vi "position_initialize.vi"(6 "Axis in":i32, 7 "New target position (units)":dbl, 9 "Velocity value (units/s)":dbl, 10 "Timeout (ms)":u32, 11 "SerialPort":u8) -> (3 "VISA Refnum out":refnum<visa-resource-name>)   [LabVIEW 2021]
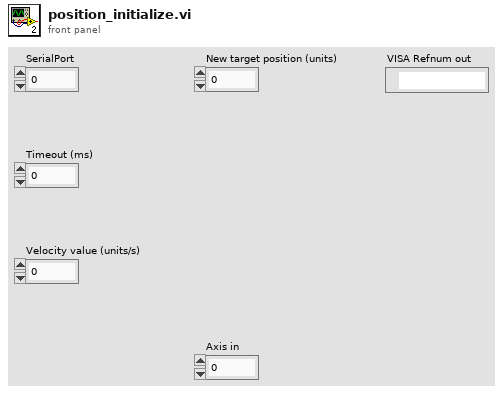
[diagram p1: front panel]
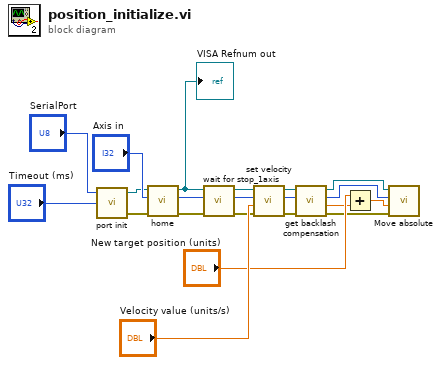
[diagram p0: block diagram]
diagram:
  n1 = call <userlib>:"port init.vi"("Timeout (ms)"="Timeout (ms)", "SerialPort"="SerialPort") -> ("error out"=w16:errorcluster, "Visa Handle"=w17:refnum<visa-resource-name>)  [unwired: 2 in]
  n2 = call <userlib>:"home.vi"("error in"=w16, "Axis in"="Axis in", "VISA Handle in"=w17) -> ("error out"=w13:errorcluster, "Axis out"=w14:i32, "VISA Handle out"=w15:refnum<visa-resource-name>)  [unwired: 3 in, 1 out]
  "VISA Refnum out" <- w15
  n3 = call <userlib>:"wait for stop_1axis.vi"("error in"=w13, "Axis in"=w14, "VISA Handle in"=w15) -> ("error out"=w10:errorcluster, "Axis out"=w11:i32, "VISA Handle out"=w12:refnum<visa-resource-name>)  [unwired: 3 in, 1 out]
  n4 = call <userlib>:"set velocity.vi"("error in"=w10, "Velocity value (units/s)"="Velocity value (units/s)", "Axis in"=w11, "VISA Handle in"=w12) -> ("error out"=w5:errorcluster, "Axis out"=w6:i32, "VISA Handle out"=w7:refnum<visa-resource-name>)  [unwired: 2 in, 1 out]
  n5 = call <userlib>:"get backlash compensation.vi"("error in"=w5, "Axis in"=w6, "VISA Handle in"=w7) -> ("error out"=w4:errorcluster, "Backlash compensation value (units)"=w8:dbl, "Axis out"=w2:i32, "VISA Handle out"=w3:refnum<visa-resource-name>)  [unwired: 2 in, 1 out]
  n6 = Add(x="New target position (units)", y=w8) -> (x+y=w1:dbl)
  n7 = call <userlib>:"Move absolute.vi"("error in"=w4, "New target position (units)"=w1, "Axis in"=w2, "VISA Handle in"=w3) -> ()  [unwired: 2 in, 4 out]
